vi "Get Test Parameters.vi"(8 "error in (no error)":errorcluster, 11 "Fiber Auto Collimation state data in":refnum<class "Fiber Auto Collimation state data.lvclass">) -> (0 "error out":errorcluster, 2 "TestParameters":T1, 3 "Fiber Auto Collimation state data out":refnum<class "Fiber Auto Collimation state data.lvclass">)   [LabVIEW 2018]
uses:
  Fiber Auto Collimation state data.lvclass
  Test Parameters.ctl
  Float keys.ctl
  String keys.ctl
  Boolean keys.ctl
  Fiber Auto Collimation state data.lvclass/Fiber Auto Collimation state data.ctl
  <userlib>/Recipe/Test Recipe classes/Test Recipe.lvclass
  C:/Program Files (x86)/National Instruments/LabVIEW 2018/user.lib/Recipe/nLight Recipe/nLight Recipe.lvclass
  <userlib>/Recipe/nLight Recipe/Look up float key.vi
  <userlib>/Recipe/nLight Recipe/Look up string key.vi
  <userlib>/Recipe/nLight Recipe/Look up boolean key.vi
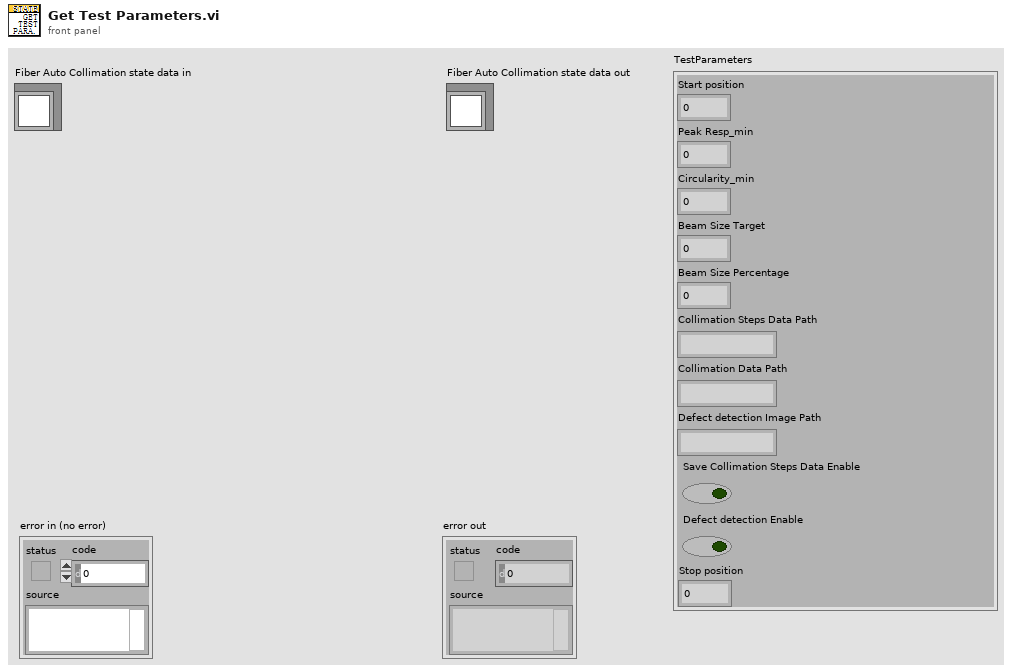
[diagram p1: front panel]
types:
  T1 = typedef "Test Parameters.ctl" = cluster{"Start position":dbl, "Peak Resp_min":dbl, "Circularity_min":dbl, "Beam Size Target":dbl, "Beam Size Percentage ":dbl, "Collimation Steps Data Path":string, "Collimation Data Path":string, "Defect detection Image Path":string, "Save Collimation Steps Data Enable":bool, "Defect detection Enable":bool, "Stop position":dbl}
  T2 = typedef "Fiber Auto Collimation state data.lvclass/Float keys.ctl" = enum16{"Start position", "Peak Resp min", "Circularity min", "Beam Size Target", "Beam Size Percentage", "Stop position"}
  T3 = typedef "Fiber Auto Collimation state data.lvclass/Boolean keys.ctl" = enum16{"Save Collimation Steps Data Enable", "Defect detection Enable"}
  T4 = typedef "Fiber Auto Collimation state data.lvclass/String keys.ctl" = enum16{"Software version", "Software name", "Collimation Steps Data Path", "Collimation Data Path", "Defect detection Image Path"}
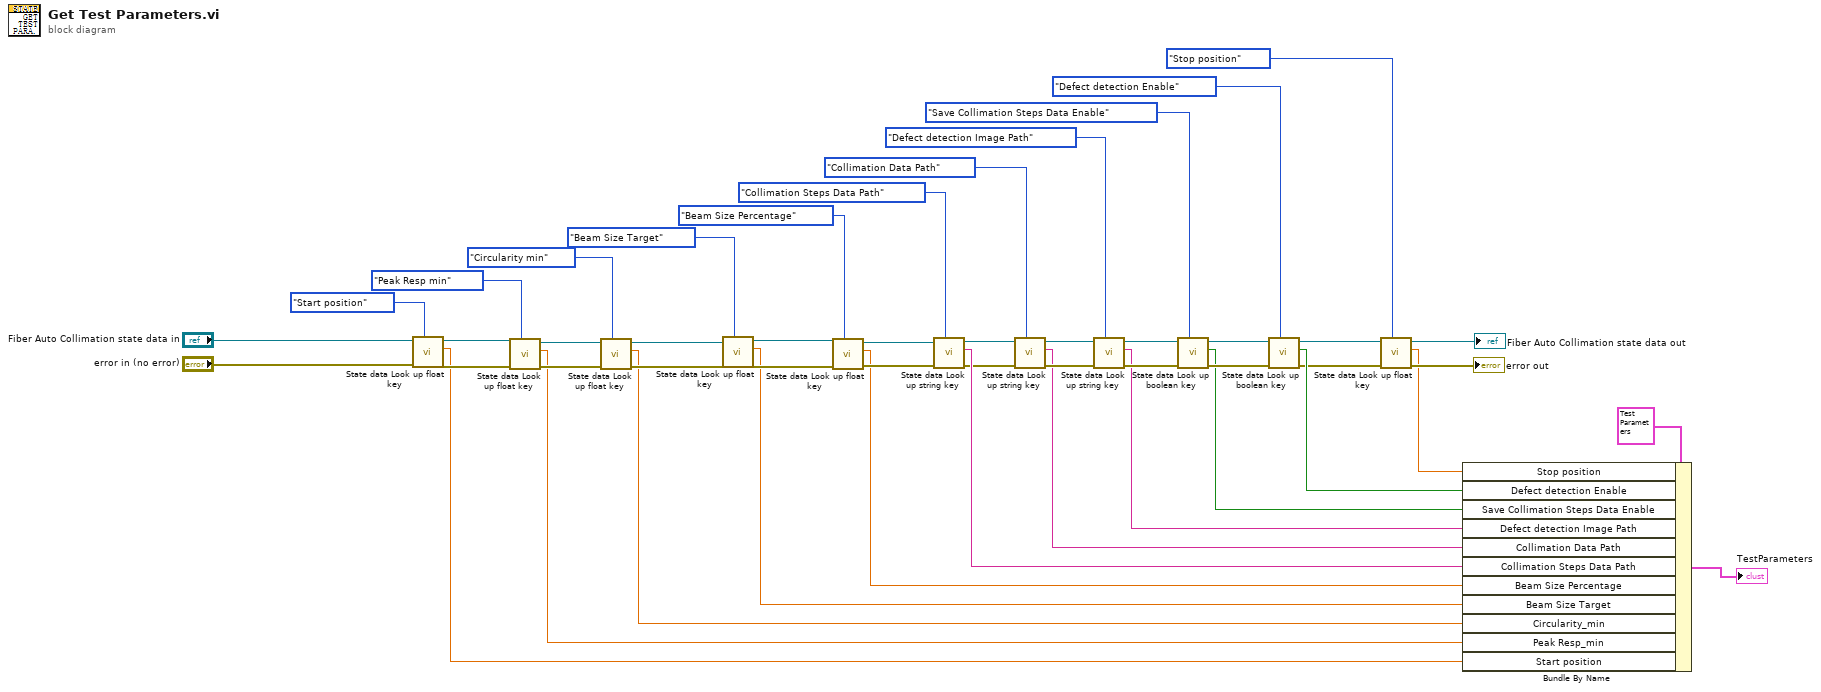
[diagram p0: block diagram]
diagram:
  n1 = call "State data Look up float key.vi"("Key [string/enum]"=Float_keys."Start position" ("Station config float keys"), "error in (no error)"="error in (no error)", "Fiber Auto Collimation state data in"="Fiber Auto Collimation state data in") -> ("error out"=w41:errorcluster, "Float Key Value"=w23:dbl, "Fiber Auto Collimation state data out"=w45:refnum<class "Fiber Auto Collimation state data.lvclass">)  [unwired: 5 in, 1 out]
  n2 = call "State data Look up float key.vi"("Key [string/enum]"=Float_keys."Peak Resp min" ("Station config float keys"), "error in (no error)"=w41, "Fiber Auto Collimation state data in"=w45) -> ("error out"=w42:errorcluster, "Float Key Value"=w24:dbl, "Fiber Auto Collimation state data out"=w43:refnum<class "Fiber Auto Collimation state data.lvclass">)  [unwired: 5 in, 1 out]
  n3 = call "State data Look up float key.vi"("Key [string/enum]"=Float_keys."Circularity min" ("Station config float keys"), "error in (no error)"=w42, "Fiber Auto Collimation state data in"=w43) -> ("error out"=w39:errorcluster, "Float Key Value"=w25:dbl, "Fiber Auto Collimation state data out"=w38:refnum<class "Fiber Auto Collimation state data.lvclass">)  [unwired: 5 in, 1 out]
  n4 = call "State data Look up float key.vi"("Key [string/enum]"=Float_keys."Beam Size Target" ("Station config float keys"), "error in (no error)"=w39, "Fiber Auto Collimation state data in"=w38) -> ("error out"=w35:errorcluster, "Float Key Value"=w26:dbl, "Fiber Auto Collimation state data out"=w36:refnum<class "Fiber Auto Collimation state data.lvclass">)  [unwired: 5 in, 1 out]
  n5 = call "State data Look up float key.vi"("Key [string/enum]"=Float_keys."Beam Size Percentage" ("Station config float keys"), "error in (no error)"=w35, "Fiber Auto Collimation state data in"=w36) -> ("error out"=w32:errorcluster, "Float Key Value"=w27:dbl, "Fiber Auto Collimation state data out"=w33:refnum<class "Fiber Auto Collimation state data.lvclass">)  [unwired: 5 in, 1 out]
  n6 = call "State data Look up string key.vi"("Key [string/enum]"=String_keys."Collimation Steps Data Path" ("Station config string keys"), "error in (no error)"=w32, "Fiber Auto Collimation state data in"=w33) -> ("error out"=w22:errorcluster, "String Key Value"=w28:string, "Fiber Auto Collimation state data out"=w15:refnum<class "Fiber Auto Collimation state data.lvclass">)  [unwired: 5 in, 1 out]
  n7 = call "State data Look up string key.vi"("Key [string/enum]"=String_keys."Collimation Data Path" ("Station config string keys"), "error in (no error)"=w22, "Fiber Auto Collimation state data in"=w15) -> ("error out"=w21:errorcluster, "String Key Value"=w14:string, "Fiber Auto Collimation state data out"=w16:refnum<class "Fiber Auto Collimation state data.lvclass">)  [unwired: 5 in, 1 out]
  n8 = call "State data Look up string key.vi"("Key [string/enum]"=String_keys."Defect detection Image Path" ("Station config string keys"), "error in (no error)"=w21, "Fiber Auto Collimation state data in"=w16) -> ("error out"=w20:errorcluster, "String Key Value"=w13:string, "Fiber Auto Collimation state data out"=w17:refnum<class "Fiber Auto Collimation state data.lvclass">)  [unwired: 5 in, 1 out]
  n9 = call "State data Look up boolean key.vi"("Key [string/enum]"=Boolean_keys."Save Collimation Steps Data Enable" ("Station config boolean keys"), "error in (no error)"=w20, "Fiber Auto Collimation state data in"=w17) -> ("error out"=w19:errorcluster, "Boolean Key Value"=w12:bool, "Fiber Auto Collimation state data out"=w18:refnum<class "Fiber Auto Collimation state data.lvclass">)  [unwired: 5 in, 1 out]
  n10 = call "State data Look up boolean key.vi"("Key [string/enum]"=Boolean_keys."Defect detection Enable" ("Station config boolean keys"), "error in (no error)"=w19, "Fiber Auto Collimation state data in"=w18) -> ("error out"=w6:errorcluster, "Boolean Key Value"=w11:bool, "Fiber Auto Collimation state data out"=w4:refnum<class "Fiber Auto Collimation state data.lvclass">)  [unwired: 5 in, 1 out]
  n11 = call "State data Look up float key.vi"("Key [string/enum]"=Float_keys."Stop position" ("Station config float keys"), "error in (no error)"=w6, "Fiber Auto Collimation state data in"=w4) -> ("error out"=→"error out":errorcluster, "Float Key Value"=w1:dbl, "Fiber Auto Collimation state data out"=→"Fiber Auto Collimation state data out":refnum<class "Fiber Auto Collimation state data.lvclass">)  [unwired: 5 in, 1 out]
  n12 = Bundle By Name(cluster=T1 {"Start position"=0.0, "Peak Resp_min"=0.0, "Circularity_min"=0.0, "Beam Size Target"=0.0, "Beam Size Percentage "=0.0, "Collimation Steps Data Path"="", "Collimation Data Path"="", "Defect detection Image Path"="", "Save Collimation Steps Data Enable"=FALSE, "Defect detection Enable"=FALSE, "Stop position"=0.0} ("TestParameters"), "Stop position"=w1, "Defect detection Enable"=w11, "Save Collimation Steps Data Enable"=w12, "Defect detection Image Path"=w13, "Collimation Data Path"=w14, "Collimation Steps Data Path"=w28, "Beam Size Percentage"=w27, "Beam Size Target"=w26, "Circularity_min"=w25, "Peak Resp_min"=w24, "Start position"=w23) -> (→"TestParameters":T1)
